vi "_f_BronkhorstLUT.vi"(6 "Delay(s)":dbl=0.075, 7 "Comunicaciones":T1={"Flujo_1"="COM4", "Brk1"=TRUE, "Flujo_2"="COM6", "Brk2"=TRUE, "Flujo_3"="COM8", "Brk3"=TRUE, "Flujo_4"="COM10", "Brk4"=TRUE, "Eurothe"="COM23", "Eurot"=FALSE, "Balanza"="COM24", "Bal"=FALSE, "eValPos"="COM25", "eVal"=FALSE, "flowbus"="COM5", "fb"=TRUE}, 8 "error in (no error)":errorcluster) -> (0 "error out":errorcluster, 3 "Dispositivos":T2=[["3", "NO", "M0000013", "Air", "1", "ln/mn", "0.1", "0.11"], ["4", "NO", "M0000014", "Air", "1", "ln/mn", "0.2", "0.22"], ["5", "NO", "M0000015", "Air", "1", "ln/mn", "0.3", "0.33"], ["6", "NO", "M0000016", "Air", "1", "ln/mn", "0.4", "0.44"], ["7", "NO", "M0000017", "Air", "1", "ln/mn", "0.5", "0.55"], ["8", "NO", "M0000018", "Air", "1", "ln/mn", "0.6", "0.66"], ["9", "NO", "M0000019", "Air", "1", "ln/mn", "0.7", "0.77"], ["10", "NO", "M0000020", "Air", "1", "ln/mn", "0.8", "0.88"], ["11", "NO", "M0000021", "Air", "1", "ln/mn", "0.9", "0.99"]] caption="Controladores de flujo FLOWBUS")   [LabVIEW 2013]
uses:
  _f_TablaBronkhorst.ctl
  Controles/P2018 Com Control.ctl
  SerialComm/_f_SerialComm_Hardware_Module Control.ctl
  _f_BronkhorstModuleControl.ctl
panel:
  out "Enable(T)":bool=TRUE
  out "VISA Bronkhorst":refnum<visa-resource-name>
  in  "stop":bool
  out "Num. of nodes":u32=6
  out "Status":string
  # "Buscando controladores"
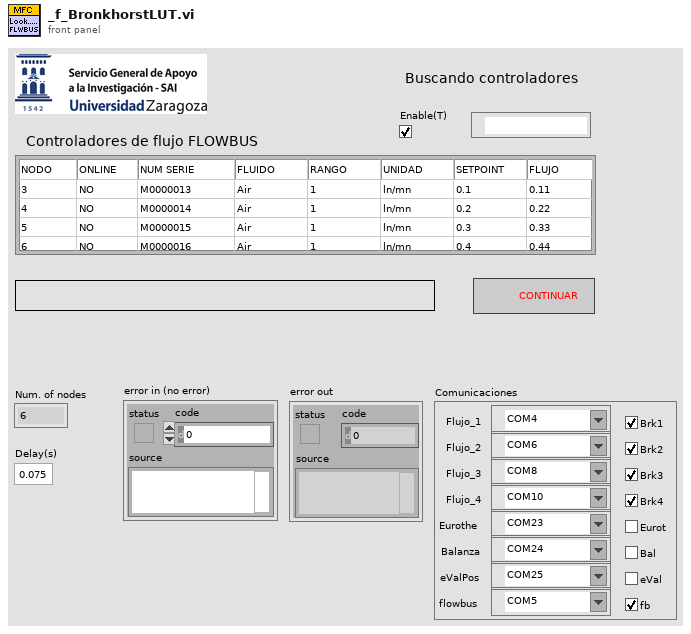
[diagram p1: front panel]
types:
  T1 = typedef "P2018 Com Control.ctl" = cluster{"Flujo_1":refnum<visa-resource-name>, "Brk1":bool, "Flujo_2":refnum<visa-resource-name>, "Brk2":bool, "Flujo_3":refnum<visa-resource-name>, "Brk3":bool, "Flujo_4":refnum<visa-resource-name>, "Brk4":bool, "Eurothe":refnum<visa-resource-name>, "Eurot":bool, "Balanza":refnum<visa-resource-name>, "Bal":bool, "eValPos":refnum<visa-resource-name>, "eVal":bool, "flowbus":refnum<visa-resource-name>, "fb":bool}
  T2 = typedef "_f_TablaBronkhorst.ctl" = string[][]
  T3 = typedef "_f_SerialComm_Hardware_Module Control.ctl" = enum16{"Initialize", "Write", "Bytes?", "Read", "Shutdown"}
  T4 = typedef "_f_BronkhorstModuleControl.ctl" = enum16{"RcharSerialNum", "RcharIdnString", "WuintFluidNum", "RuintFluidNum", "RcharFluidName", "RuintSensorType", "RfloatCap0", "RfloatCap100", "RcharCapUnitStr", "W%Setpoint", "R%Setpoint", "R%Measure", "WfloatSetpoint", "RfloatSetpoint", "RfloatMeasure ", "RfloatDensity", "WuintControlMode", "WcharRESET", "RfloatCounter", "RcharCounterUnit", "WfloatCounterLimit", "RfloatCounterLimit", "WcharCounterMode", "RcharCounterMode", "WcharCounterSPMode", "RcharCounterSPMode", "WcharCounterNewSP", "RcharCounterNewSP"}
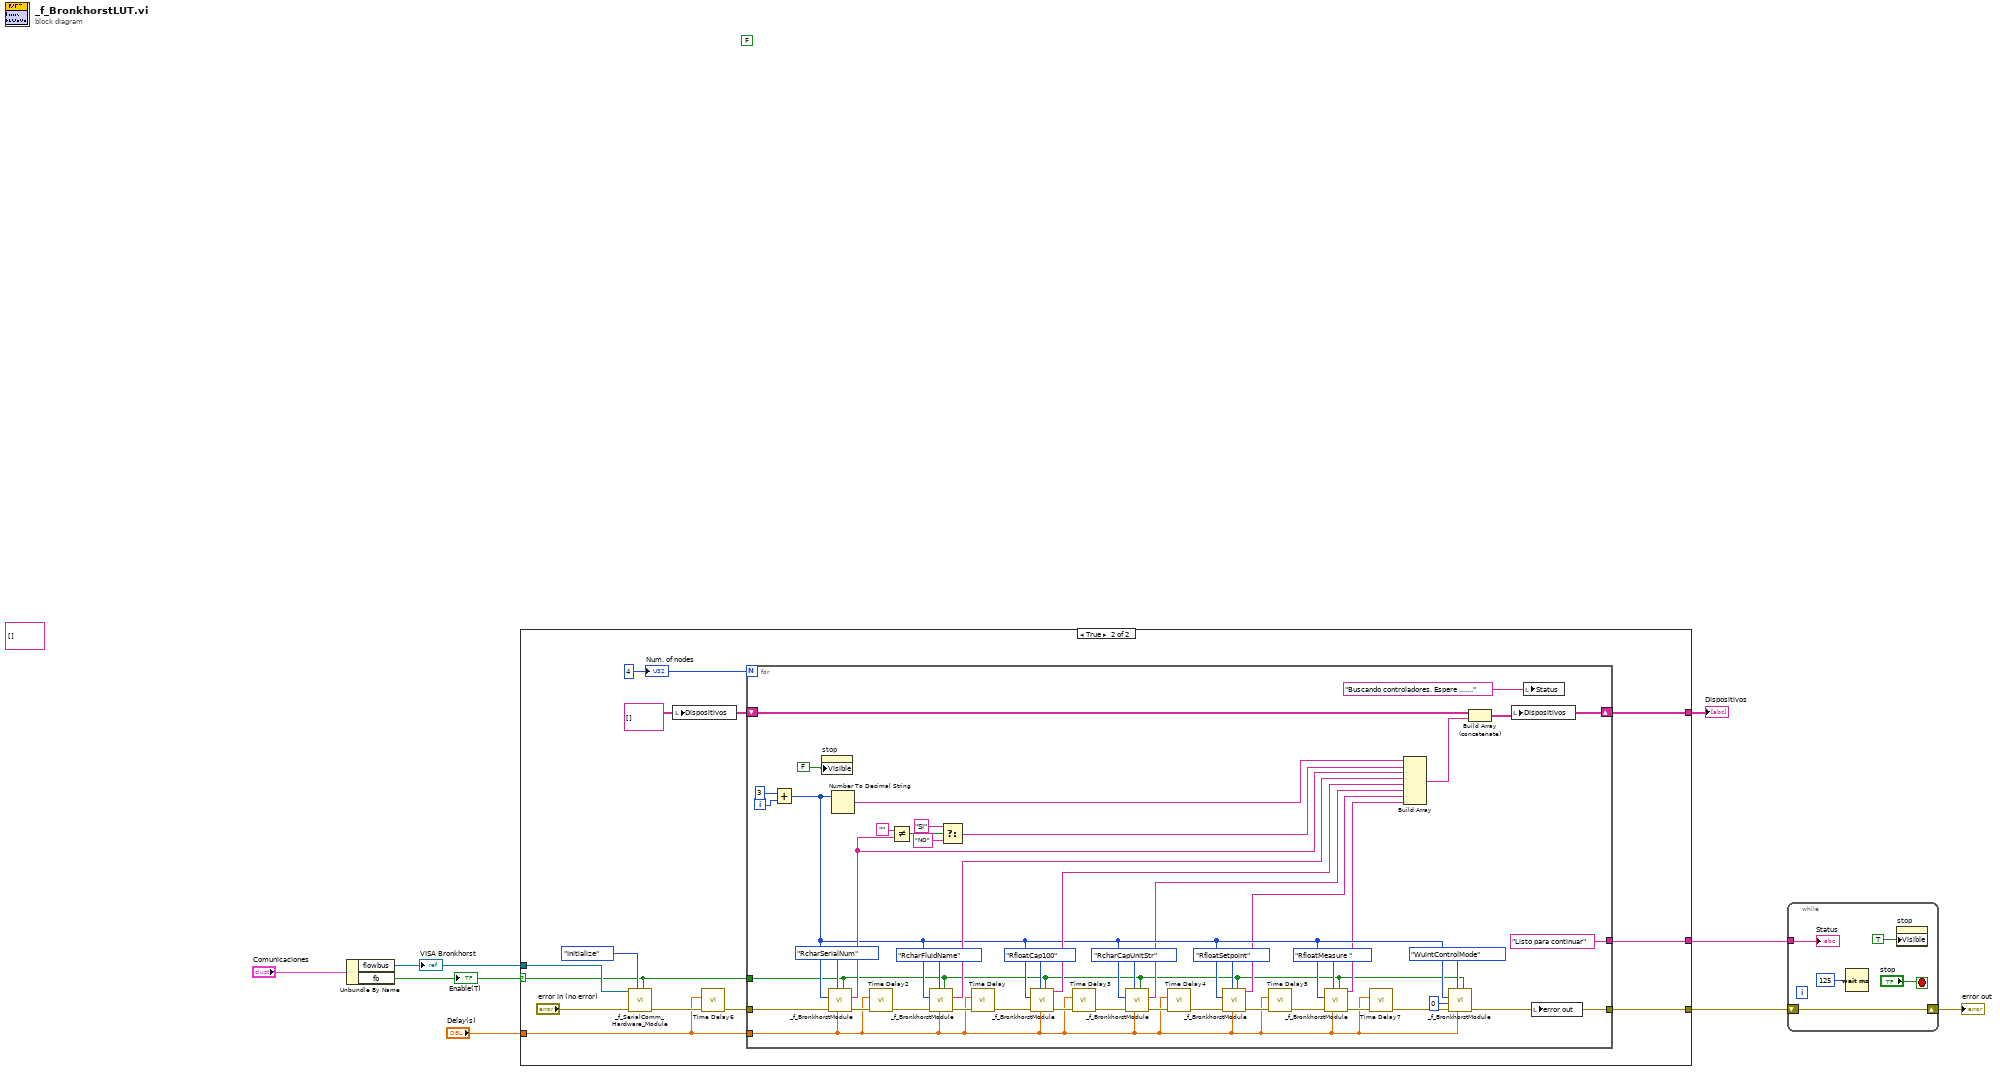
[diagram p0: block diagram]
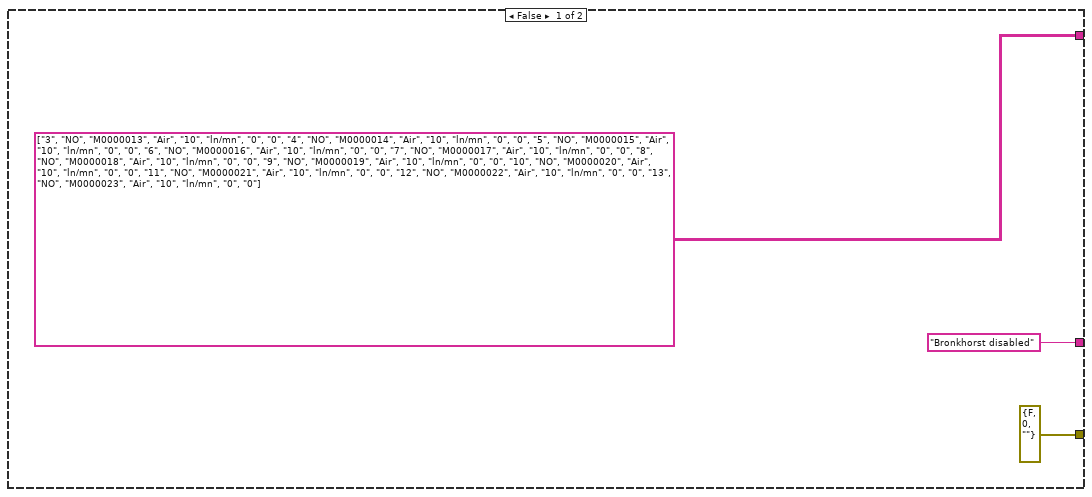
[diagram p2: hidden frame]
diagram:
  (unwired) string[][] []
  (unwired) FALSE
  n1 = Unbundle By Name("Comunicaciones") -> ("flowbus"=w4:refnum<visa-resource-name>, "fb"=w5:bool)
  "Enable(T)" <- w5
  "VISA Bronkhorst" <- w4
  n2 = case shown="True" w5 {
    selector: w5 -> [_ w12]
    tunnel: w4 -> [_ w23]
    tunnel: [T2 [["3", "NO", "M0000013", "Air", "10", "ln/mn", "0", "0"], ["4", "NO", "M0000014", "Air", "10", "ln/mn", "0", "0"], ["5", "NO", "M0000015", "Air", "10", "ln/mn", "0", "0"], ["6", "NO", "M0000016", "Air", "10", "ln/mn", "0", "0"], ["7", "NO", "M0000017", "Air", "10", "ln/mn", "0", "0"], ["8", "NO", "M0000018", "Air", "10", "ln/mn", "0", "0"], ["9", "NO", "M0000019", "Air", "10", "ln/mn", "0", "0"], ["10", "NO", "M0000020", "Air", "10", "ln/mn", "0", "0"], ["11", "NO", "M0000021", "Air", "10", "ln/mn", "0", "0"], ["12", "NO", "M0000022", "Air", "10", "ln/mn", "0", "0"], ["13", "NO", "M0000023", "Air", "10", "ln/mn", "0", "0"]] ("Dispositivos") w21] -> w3
    tunnel: ["Bronkhorst disabled" ("Status") w15] -> w8
    tunnel: [errorcluster {"status"=FALSE, "code"=0, "source"=""} ("error out") w14] -> w6
    tunnel: "Delay(s)" -> [_ w13]
    frame False {
    }
    frame True {
      w19 = 4 ("Nodos 2")
      w22 = string[][] []
      n3 = call "_f_SerialComm_Hardware_Module.vi"("Enable(T)"=w12, "Command"=_f_SerialComm_Hardware_Module_Control."Initialize", "error in (no error)"="error in (no error)", "VISA resource name"=w23) -> ("error out"=w18:errorcluster)  [unwired: 5 in, 2 out]
      n4 = local write "Dispositivos"(w22) -> ()
      n5 = call "Time Delay6"("error in (no error)"=w18, "Delay Time (s)"=w13) -> ("error out"=w17:errorcluster)  [unwired: 9 in]
      n6 = for {
        N: w19 -> [_]
        tunnel: w17 -> [w40]
        tunnel: [w38] -> w14
        tunnel: w13 -> [w27]
        shift-right: [w46] -> w21
        shift-left: w22 -> [w50]
        tunnel: ["Listo para continuar" ("Status")] -> w15
        tunnel: w12 -> [w24]
        i -> [w66]
        n7 = Add(x=3, y=w66) -> (x+y=w31:i32)
        n8 = property on="stop" class="Bool"("Visible"=FALSE) -> ()  [unwired: 2 in, 2 out]
        n9 = call "_f_BronkhorstModule.vi"("Enable(T)"=w24, "Delay"=w27, "Command"=_f_BronkhorstModuleControl."RcharSerialNum", "error in (no error)"=w40, "Nodo"=w31) -> ("error out"=w62:errorcluster, "Result"=w41:string)  [unwired: 3 in, 2 out]
        n10 = Number To Decimal String(number=w31) -> (decimal integer string=w47:string)  [unwired: 1 in]
        n11 = call "Time Delay2"("error in (no error)"=w62, "Delay Time (s)"=w27) -> ("error out"=w61:errorcluster)  [unwired: 9 in]
        n12 = Not Equal?(x="", y=w41) -> (x != y?=w58:bool)
        n13 = call "_f_BronkhorstModule.vi"("Enable(T)"=w24, "Delay"=w27, "Command"=_f_BronkhorstModuleControl."RcharFluidName", "error in (no error)"=w61, "Nodo"=w31) -> ("error out"=w60:errorcluster, "Result"=w48:string)  [unwired: 3 in, 2 out]
        n14 = Select(t="SI", s=w58, f="NO") -> (s? t:f=w51:string)
        n15 = call "Time Delay"("error in (no error)"=w60, "Delay Time (s)"=w27) -> ("error out"=w55:errorcluster)  [unwired: 9 in]
        n16 = call "_f_BronkhorstModule.vi"("Enable(T)"=w24, "Delay"=w27, "Command"=_f_BronkhorstModuleControl."RfloatCap100", "error in (no error)"=w55, "Nodo"=w31) -> ("error out"=w52:errorcluster, "Value"=w42:string)  [unwired: 3 in, 2 out]
        n17 = call "Time Delay3"("error in (no error)"=w52, "Delay Time (s)"=w27) -> ("error out"=w53:errorcluster)  [unwired: 9 in]
        n18 = call "_f_BronkhorstModule.vi"("Enable(T)"=w24, "Delay"=w27, "Command"=_f_BronkhorstModuleControl."RcharCapUnitStr", "error in (no error)"=w53, "Nodo"=w31) -> ("error out"=w54:errorcluster, "Result"=w30:string)  [unwired: 3 in, 2 out]
        n19 = call "Time Delay4"("error in (no error)"=w54, "Delay Time (s)"=w27) -> ("error out"=w43:errorcluster)  [unwired: 9 in]
        n20 = call "_f_BronkhorstModule.vi"("Enable(T)"=w24, "Delay"=w27, "Command"=_f_BronkhorstModuleControl."RfloatSetpoint", "error in (no error)"=w43, "Nodo"=w31) -> ("error out"=w36:errorcluster, "Value"=w28:string)  [unwired: 3 in, 2 out]
        n21 = call "Time Delay5"("error in (no error)"=w36, "Delay Time (s)"=w27) -> ("error out"=w33:errorcluster)  [unwired: 9 in]
        n22 = call "_f_BronkhorstModule.vi"("Enable(T)"=w24, "Delay"=w27, "Command"=_f_BronkhorstModuleControl."RfloatMeasure ", "error in (no error)"=w33, "Nodo"=w31) -> ("error out"=w34:errorcluster, "Value"=w29:string)  [unwired: 3 in, 2 out]
        n23 = call "Time Delay7"("error in (no error)"=w34, "Delay Time (s)"=w27) -> ("error out"=w32:errorcluster)  [unwired: 9 in]
        n24 = Build Array(w47, w51, w41, w48, w42, w30, w28, w29) -> (w49:string[])
        n25 = call "_f_BronkhorstModule.vi"("Enable(T)"=w24, "Delay"=w27, "Command"=_f_BronkhorstModuleControl."WuintControlMode", "error in (no error)"=w32, "Value"=0 ("x"), "Nodo"=w31) -> ("error out"=w38:errorcluster)  [unwired: 2 in, 3 out]
        n26 = Build Array (concatenate)(w50, w49) -> (w46:string[][])
        n27 = local write "Dispositivos"(w46) -> ()
        n28 = local write "Status"("Buscando controladores. Espere ......." ("Status")) -> ()
        n29 = local write "error out"(w38) -> ()
      }
      "Num. of nodes" <- w19
    }
  }
  "Dispositivos" <- w3
  n30 = while {
    tunnel: w8 -> [w71]
    shift-right: [w69] -> w7
    shift-left: w6 -> [w69]
    stop <- "stop" stop-if-true
    n31 = Wait (ms)(milliseconds to wait=u32 125) -> ()  [unwired: 1 out]
    n32 = property on="stop" class="Bool"("Visible"=TRUE) -> ()  [unwired: 2 in, 2 out]
    "Status" <- w71
  }
  "error out" <- w7
